vi "To String.vi"(8 "error in (no error)":errorcluster, 11 "Enum in":refnum<class "Enum.lvclass">) -> (0 "error out":errorcluster, 2 "String":string)   [LabVIEW 2020, in "Data.lvlib" / "Enum.lvclass"]
doc: "Convert 'Generic Data in' to a string."
uses:
  Enum.lvclass
  Enum.lvclass/Enum.ctl
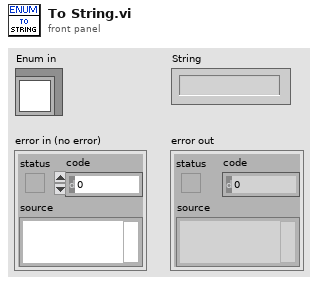
[diagram p1: front panel]
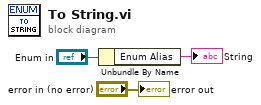
[diagram p0: block diagram]
diagram:
  n1 = Unbundle By Name("Enum in") -> ("Enum Alias"=→"String":string)
  "error out" <- "error in (no error)"
